vi "Flowmeter Final.vi"() -> ()   [LabVIEW 2018]
panel:
  in  "Induced EMF 5 (mV)":dbl(knob) scale=0.0..10.0
  in  "Induced EMF 4 (mV)":dbl(knob) scale=0.0..10.0
  in  "Induced EMF 3 (mV)":dbl(knob) scale=0.0..10.0
  in  "Induced EMF 2 (mV)":dbl(knob) scale=0.0..10.0
  in  "Electromagnetic Flow Meter Graphs":u16(ring) items=["EMF Induced", "Magnetic FIeld", "Diameter of Pipe"]
  in  "Doppler Flow Meter Graphs":u16(ring) items=["Ultrasound Speed", "Theta", "Frequency"]
  in  "Speed of Sound in Fluid (m/s)":dbl(knob) scale=0.0..1000.0
  out "XY Graph":cluster{"Y":dbl[], "Y":dbl[]}[](graph)
  in  "Switch 2":bool
  out "?":bool
  out "Velocity":dbl(knob) scale=0.0..1000.0
  in  "Ultrasonic Mode Switch":bool
  in  "?":bool
  in  "Thickness of pipe (mm)":dbl(slide) scale=0.0..1000.0
  in  "Magnetic Field (mT)":dbl(knob) scale=0.0..1000.0
  in  "Induced EMF 1 (mV)":dbl(knob) scale=0.0..10.0
  in  "Angle":dbl(knob) scale=90.0..30.0
  in  "Frequency 1 (KHz)":dbl(knob) scale=0.0..1000.0
  in  "Frequency 2 (KHz)":dbl(knob) scale=0.0..1000.0
  in  "milliseconds to wait":dbl
  in  "?":bool
  # "Variation wrt Difference\n      in Frequency"
  # "Variation wrt Angle"
  # "Electromagnetic"
  # "Ultrasonic"
  # "Doppler Flow Meter"
  # "Transit Time"
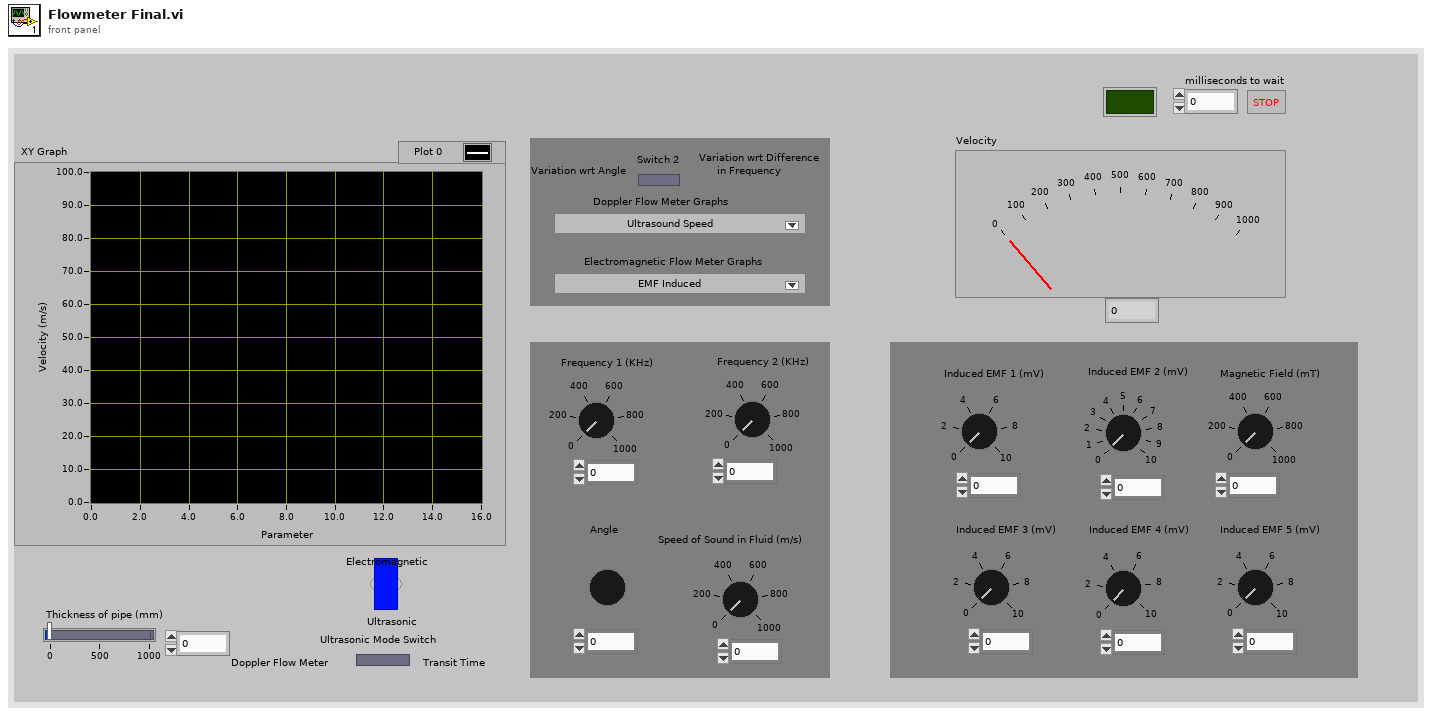
[diagram p1: front panel]
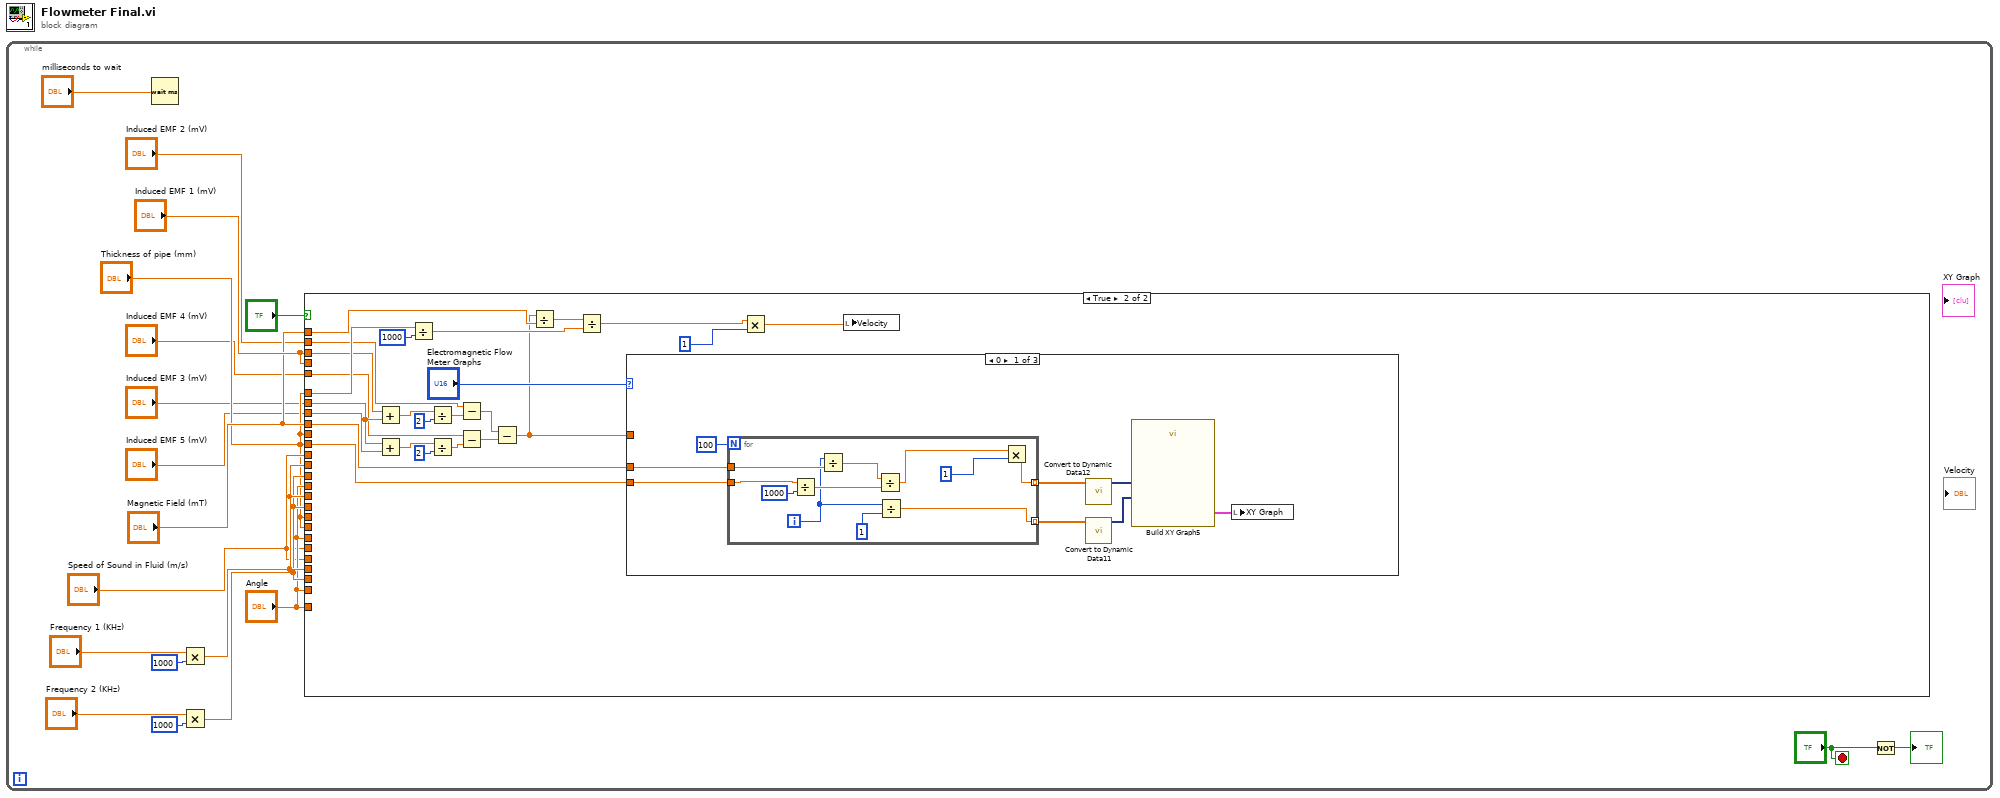
[diagram p0: block diagram]
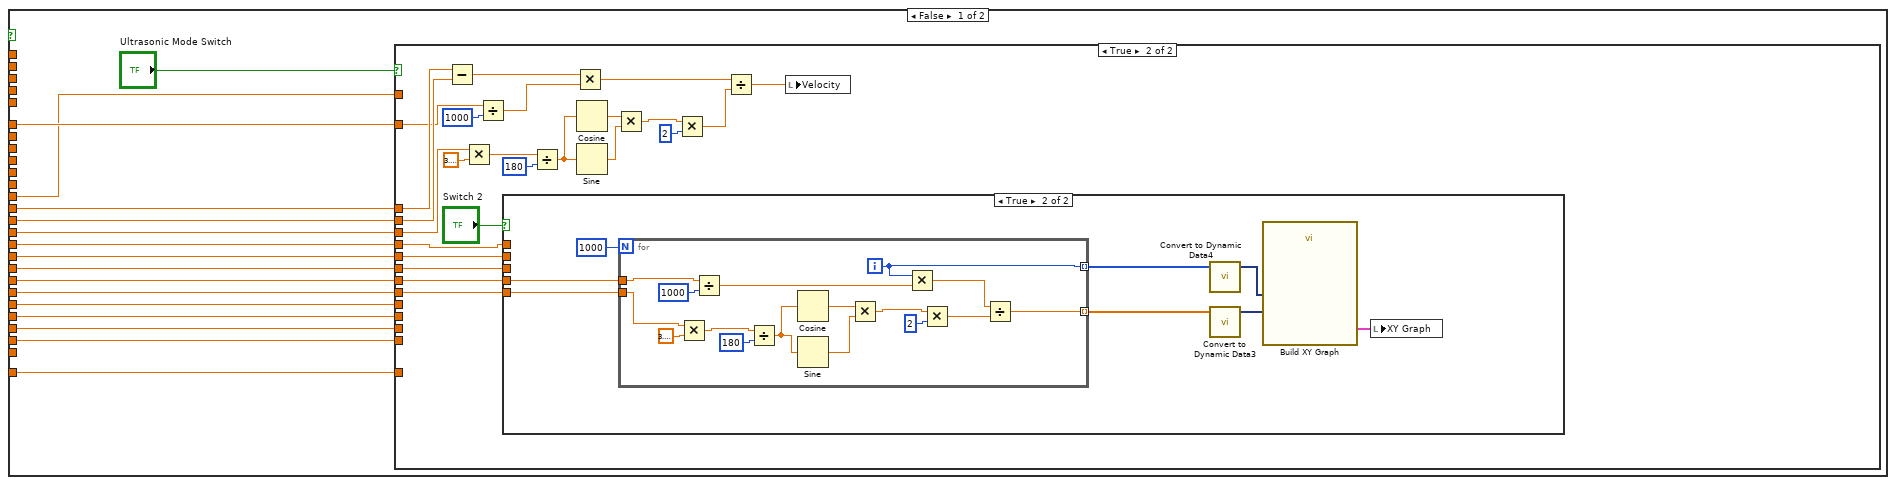
[diagram p2: hidden frame]
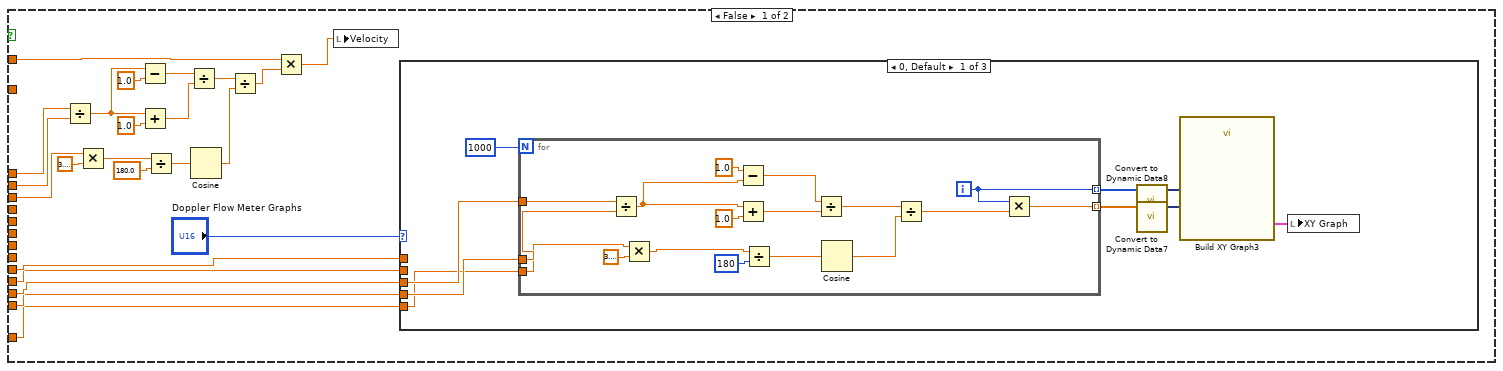
[diagram p3: hidden frame]
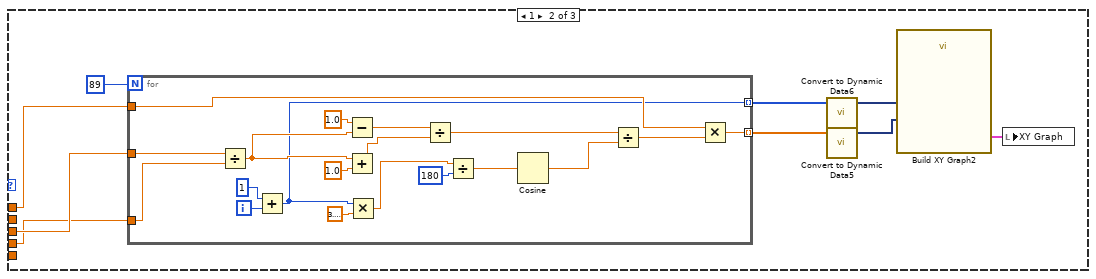
[diagram p4: hidden frame]
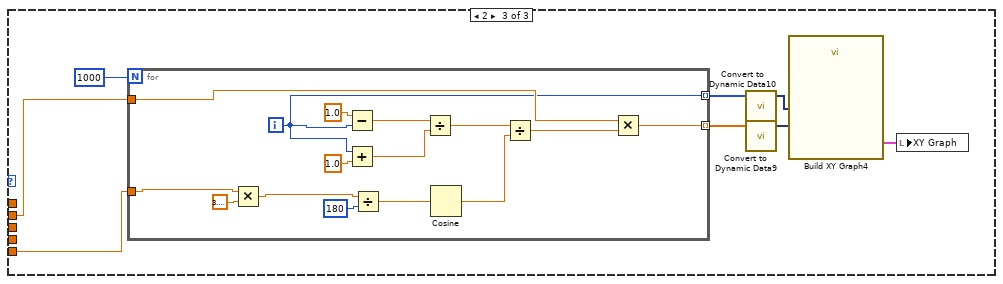
[diagram p5: hidden frame]
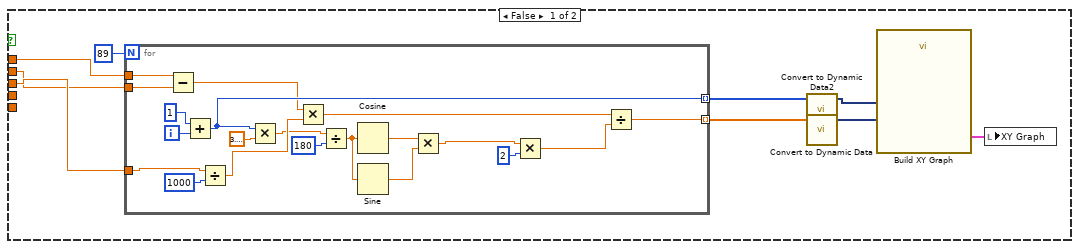
[diagram p6: hidden frame]
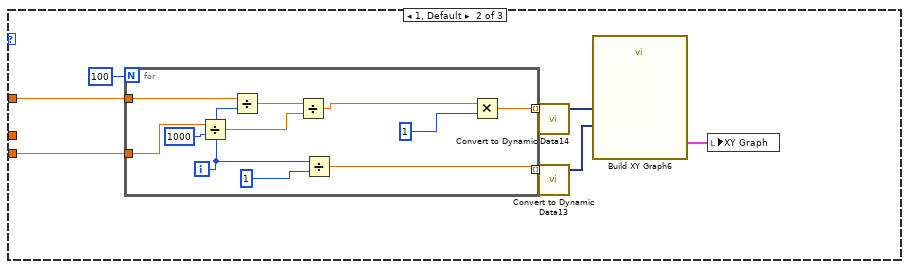
[diagram p7: hidden frame]
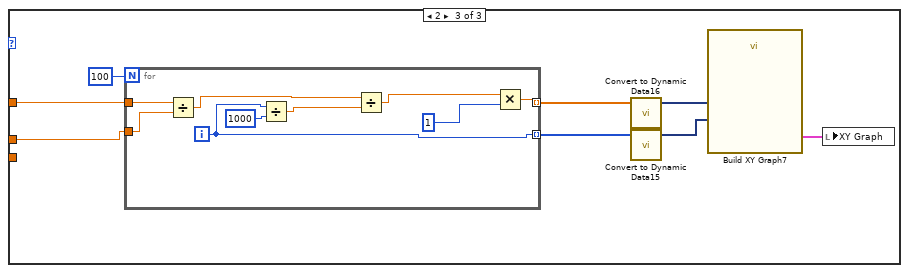
[diagram p8: hidden frame]
diagram:
  n1 = while {
    stop <- "?" stop-if-true
    n2 = Wait (ms)(milliseconds to wait="milliseconds to wait") -> ()  [unwired: 1 out]
    n3 = Multiply(x="Frequency 1 (KHz)", y=1000) -> (x*y=w11:dbl)
    n4 = Multiply(x="Frequency 2 (KHz)", y=1000) -> (x*y=w10:dbl)
    n5 = case shown="True" "?" {
      tunnel: "Angle" -> [w32 _]
      tunnel: "Thickness of pipe (mm)" -> [w33 w235]
      tunnel: w10 -> [w34 _]
      tunnel: w11 -> [w35 _]
      tunnel: "Angle" -> [_ _]
      tunnel: "Thickness of pipe (mm)" -> [_ _]
      tunnel: "Thickness of pipe (mm)" -> [w29 _]
      tunnel: w11 -> [w31 _]
      tunnel: w10 -> [w30 _]
      tunnel: "Induced EMF 1 (mV)" -> [_ w229]
      tunnel: "Magnetic Field (mT)" -> [_ w236]
      tunnel: "Thickness of pipe (mm)" -> [w27 _]
      tunnel: "Angle" -> [w26 _]
      tunnel: "Speed of Sound in Fluid (m/s)" -> [w25 _]
      tunnel: w11 -> [w24 _]
      tunnel: w10 -> [w23 _]
      tunnel: "Speed of Sound in Fluid (m/s)" -> [w22 _]
      tunnel: "Angle" -> [w21 _]
      tunnel: "Speed of Sound in Fluid (m/s)" -> [w20 _]
      tunnel: "Induced EMF 1 (mV)" -> [_ _]
      tunnel: "Magnetic Field (mT)" -> [_ w232]
      tunnel: "Thickness of pipe (mm)" -> [_ w231]
      tunnel: "Induced EMF 2 (mV)" -> [_ w220]
      tunnel: "Induced EMF 3 (mV)" -> [_ w228]
      tunnel: "Induced EMF 5 (mV)" -> [_ w227]
      tunnel: "Induced EMF 4 (mV)" -> [_ w219]
      frame False {
        n6 = case shown="True" "Ultrasonic Mode Switch" {
          tunnel: w35 -> [w46 w146]
          tunnel: w34 -> [w45 w145]
          tunnel: w33 -> [_ w144]
          tunnel: w32 -> [w44 w143]
          tunnel: w31 -> [_ w142]
          tunnel: w30 -> [_ w141]
          tunnel: w29 -> [_ w140]
          tunnel: w27 -> [_ w138]
          tunnel: w26 -> [_ w137]
          tunnel: w25 -> [w43 _]
          tunnel: w24 -> [w40 _]
          tunnel: w23 -> [w39 _]
          tunnel: w22 -> [w38 _]
          tunnel: w21 -> [w37 _]
          tunnel: w20 -> [w36 _]
          frame False {
            n7 = Divide(x=w46, y=w45) -> (x/y=w48:dbl)
            n8 = Multiply(x=w44, y=3.141592653589793) -> (x*y=w52:dbl)
            n9 = Subtract(x=w48, y=1.0 ("x")) -> (x-y=w57:dbl)
            n10 = Add(x=w48, y=1.0) -> (x+y=w56:dbl)
            n11 = Divide(x=w52, y=180.0) -> (x/y=w51:dbl)
            n12 = Divide(x=w57, y=w56) -> (x/y=w55:dbl)
            n13 = Cosine(x=w51) -> (cos(x)=w53:dbl)
            n14 = Divide(x=w55, y=w53) -> (x/y=w54:dbl)
            n15 = Multiply(x=w43, y=w54) -> (x*y=w42:dbl)
            n16 = local write "Velocity"(w42) -> ()
            n17 = case shown="0, Default" "Doppler Flow Meter Graphs" {
              tunnel: w40 -> [w62 w92 _]
              tunnel: w39 -> [w61 w91 _]
              tunnel: w38 -> [_ w90 _]
              tunnel: w37 -> [w60 _ w115]
              tunnel: w36 -> [_ _ w114]
              frame 0, Default {
                n18 = for {
                  N: 1000 -> [_]
                  tunnel: w62 -> [w77]
                  tunnel: w61 -> [w76]
                  tunnel: [w75] -> w63 mode=indexing
                  tunnel: [w68] -> w64 mode=indexing
                  tunnel: w60 -> [w69]
                  i -> [w68]
                  n19 = Divide(x=w77, y=w76) -> (x/y=w70:dbl)
                  n20 = Multiply(x=w69, y=3.141592653589793) -> (x*y=w74:dbl)
                  n21 = Subtract(x=1.0, y=w70) -> (x-y=w82:dbl)
                  n22 = Add(x=w70, y=1.0) -> (x+y=w81:dbl)
                  n23 = Divide(x=w74, y=180) -> (x/y=w71:dbl)
                  n24 = Divide(x=w82, y=w81) -> (x/y=w80:dbl)
                  n25 = Cosine(x=w71) -> (cos(x)=w78:dbl)
                  n26 = Divide(x=w80, y=w78) -> (x/y=w79:dbl)
                  n27 = Multiply(x=w68, y=w79) -> (x*y=w75:dbl)
                }
                n28 = call "Convert to Dynamic Data8"("Array"=w64) -> ("Dynamic Data Type"=w66:dynamicdata)  [unwired: 3 in]
                n29 = call "Convert to Dynamic Data7"("Array"=w63) -> ("Dynamic Data Type"=w65:dynamicdata)  [unwired: 3 in]
                n30 = call "Build XY Graph3"("Y Input"=w65, "X Input"=w66) -> ("XY Graph"=w59:cluster{"X":dbl[], "Y":dbl[]}[])  [unwired: 8 in, 1 out]
                n31 = local write "XY Graph"(w59) -> ()
              }
              frame 1 {
                n32 = for {
                  N: 89 -> [_]
                  tunnel: w92 -> [w105]
                  tunnel: w91 -> [w104]
                  tunnel: [w103] -> w86 mode=indexing
                  tunnel: [w94] -> w87 mode=indexing
                  tunnel: w90 -> [w95]
                  i -> [w102]
                  n33 = Divide(x=w105, y=w104) -> (x/y=w96:dbl)
                  n34 = Add(x=1, y=w102) -> (x+y=w94:i32)
                  n35 = Subtract(x=1.0, y=w96) -> (x-y=w110:dbl)
                  n36 = Add(x=w96, y=1.0) -> (x+y=w109:dbl)
                  n37 = Multiply(x=w94, y=3.141592653589793) -> (x*y=w100:dbl)
                  n38 = Divide(x=w110, y=w109) -> (x/y=w108:dbl)
                  n39 = Divide(x=w100, y=180) -> (x/y=w97:dbl)
                  n40 = Cosine(x=w97) -> (cos(x)=w106:dbl)
                  n41 = Divide(x=w108, y=w106) -> (x/y=w107:dbl)
                  n42 = Multiply(x=w95, y=w107) -> (x*y=w103:dbl)
                }
                n43 = call "Convert to Dynamic Data6"("Array"=w87) -> ("Dynamic Data Type"=w89:dynamicdata)  [unwired: 3 in]
                n44 = call "Convert to Dynamic Data5"("Array"=w86) -> ("Dynamic Data Type"=w88:dynamicdata)  [unwired: 3 in]
                n45 = call "Build XY Graph2"("Y Input"=w88, "X Input"=w89) -> ("XY Graph"=w85:cluster{"X":dbl[], "Y":dbl[]}[])  [unwired: 8 in, 1 out]
                n46 = local write "XY Graph"(w85) -> ()
              }
              frame 2 {
                n47 = for {
                  N: 1000 -> [_]
                  tunnel: [w128] -> w116 mode=indexing
                  tunnel: [w121] -> w117 mode=indexing
                  tunnel: w115 -> [w123]
                  tunnel: w114 -> [w122]
                  i -> [w121]
                  n48 = Multiply(x=w123, y=3.141592653589793) -> (x*y=w127:dbl)
                  n49 = Subtract(x=1.0, y=w121) -> (x-y=w133:dbl)
                  n50 = Add(x=w121, y=1.0) -> (x+y=w132:dbl)
                  n51 = Divide(x=w127, y=180) -> (x/y=w124:dbl)
                  n52 = Divide(x=w133, y=w132) -> (x/y=w131:dbl)
                  n53 = Cosine(x=w124) -> (cos(x)=w129:dbl)
                  n54 = Divide(x=w131, y=w129) -> (x/y=w130:dbl)
                  n55 = Multiply(x=w122, y=w130) -> (x*y=w128:dbl)
                }
                n56 = call "Convert to Dynamic Data10"("Array"=w117) -> ("Dynamic Data Type"=w119:dynamicdata)  [unwired: 3 in]
                n57 = call "Convert to Dynamic Data9"("Array"=w116) -> ("Dynamic Data Type"=w118:dynamicdata)  [unwired: 3 in]
                n58 = call "Build XY Graph4"("Y Input"=w118, "X Input"=w119) -> ("XY Graph"=w113:cluster{"X":dbl[], "Y":dbl[]}[])  [unwired: 8 in, 1 out]
                n59 = local write "XY Graph"(w113) -> ()
              }
            }
          }
          frame True {
            n60 = Subtract(x=w146, y=w145) -> (x-y=w147:dbl)
            n61 = Multiply(x=w143, y=3.141592653589793) -> (x*y=w157:dbl)
            n62 = Divide(x=w144, y=1000) -> (x/y=w148:dbl)
            n63 = case shown="True" "Switch 2" {
              tunnel: w137 -> [_ w191]
              tunnel: w138 -> [_ w190]
              tunnel: w140 -> [w163 _]
              tunnel: w142 -> [w162 _]
              tunnel: w141 -> [w161 _]
              frame False {
                n64 = for {
                  N: 89 -> [_]
                  tunnel: w163 -> [w176]
                  tunnel: w162 -> [w174]
                  tunnel: [w170] -> w164 mode=indexing
                  tunnel: [w175] -> w165 mode=indexing
                  tunnel: w161 -> [w173]
                  i -> [w172]
                  n65 = Subtract(x=w174, y=w173) -> (x-y=w169:dbl)
                  n66 = Add(x=1, y=w172) -> (x+y=w170:i32)
                  n67 = Divide(x=w176, y=1000) -> (x/y=w188:dbl)
                  n68 = Multiply(x=w170, y=3.141592653589793) -> (x*y=w181:dbl)
                  n69 = Multiply(x=w169, y=w188) -> (x*y=w186:dbl)
                  n70 = Divide(x=w181, y=180) -> (x/y=w182:dbl)
                  n71 = Cosine(x=w182) -> (cos(x)=w183:dbl)
                  n72 = Sine(x=w182) -> (sin(x)=w184:dbl)
                  n73 = Multiply(x=w183, y=w184) -> (x*y=w185:dbl)
                  n74 = Multiply(x=w185, y=2) -> (x*y=w187:dbl)
                  n75 = Divide(x=w186, y=w187) -> (x/y=w175:dbl)
                }
                n76 = call "Convert to Dynamic Data2"("Array"=w164) -> ("Dynamic Data Type"=w166:dynamicdata)  [unwired: 3 in]
                n77 = call "Convert to Dynamic Data"("Array"=w165) -> ("Dynamic Data Type"=w167:dynamicdata)  [unwired: 3 in]
                n78 = call "Build XY Graph"("Y Input"=w167, "X Input"=w166) -> ("XY Graph"=w160:cluster{"X":dbl[], "Y":dbl[]}[])  [unwired: 8 in, 1 out]
                n79 = local write "XY Graph"(w160) -> ()
              }
              frame True {
                n80 = for {
                  N: 1000 -> [_]
                  tunnel: w190 -> [w200]
                  tunnel: w191 -> [w199]
                  tunnel: [w197] -> w192 mode=indexing
                  tunnel: [w198] -> w193 mode=indexing
                  i -> [w197]
                  n81 = Multiply(x=w199, y=3.141592653589793) -> (x*y=w205:dbl)
                  n82 = Divide(x=w200, y=1000) -> (x/y=w212:dbl)
                  n83 = Divide(x=w205, y=180) -> (x/y=w206:dbl)
                  n84 = Cosine(x=w206) -> (cos(x)=w207:dbl)
                  n85 = Sine(x=w206) -> (sin(x)=w208:dbl)
                  n86 = Multiply(x=w207, y=w208) -> (x*y=w209:dbl)
                  n87 = Multiply(x=w197, y=w212) -> (x*y=w210:dbl)
                  n88 = Multiply(x=w209, y=2) -> (x*y=w211:dbl)
                  n89 = Divide(x=w210, y=w211) -> (x/y=w198:dbl)
                }
                n90 = call "Convert to Dynamic Data4"("Array"=w192) -> ("Dynamic Data Type"=w194:dynamicdata)  [unwired: 3 in]
                n91 = call "Convert to Dynamic Data3"("Array"=w193) -> ("Dynamic Data Type"=w195:dynamicdata)  [unwired: 3 in]
                n92 = call "Build XY Graph"("Y Input"=w195, "X Input"=w194) -> ("XY Graph"=w189:cluster{"X":dbl[], "Y":dbl[]}[])  [unwired: 8 in, 1 out]
                n93 = local write "XY Graph"(w189) -> ()
              }
            }
            n94 = Divide(x=w157, y=180) -> (x/y=w155:dbl)
            n95 = Multiply(x=w147, y=w148) -> (x*y=w151:dbl)
            n96 = Cosine(x=w155) -> (cos(x)=w154:dbl)
            n97 = Sine(x=w155) -> (sin(x)=w153:dbl)
            n98 = Multiply(x=w154, y=w153) -> (x*y=w152:dbl)
            n99 = Multiply(x=w152, y=2) -> (x*y=w150:dbl)
            n100 = Divide(x=w151, y=w150) -> (x/y=w136:dbl)
            n101 = local write "Velocity"(w136) -> ()
          }
        }
      }
      frame True {
        n102 = Add(x=w229, y=w228) -> (x+y=w226:dbl)
        n103 = Add(x=w228, y=w227) -> (x+y=w225:dbl)
        n104 = Divide(x=w235, y=1000) -> (x/y=w233:dbl)
        n105 = Divide(x=w226, y=2) -> (x/y=w224:dbl)
        n106 = Divide(x=w225, y=2) -> (x/y=w223:dbl)
        n107 = Subtract(x=w220, y=w224) -> (x-y=w217:dbl)
        n108 = Subtract(x=w219, y=w223) -> (x-y=w216:dbl)
        n109 = Subtract(x=w217, y=w216) -> (x-y=w218:dbl)
        n110 = Divide(x=w218, y=w236) -> (x/y=w234:dbl)
        n111 = Divide(x=w234, y=w233) -> (x/y=w215:dbl)
        n112 = case shown="0" "Electromagnetic Flow Meter Graphs" {
          tunnel: w218 -> [_ w260 w279]
          tunnel: w232 -> [w245 _ w278]
          tunnel: w231 -> [w240 w259 _]
          frame 0 {
            n113 = for {
              N: 100 -> [_]
              tunnel: [w250] -> w242 mode=indexing
              tunnel: w245 -> [w253]
              tunnel: [w246] -> w241 mode=indexing
              tunnel: w240 -> [w252]
              i -> [w247]
              n114 = Divide(x=w252, y=1000) -> (x/y=w254:dbl)
              n115 = Divide(x=w247, y=w253) -> (x/y=w255:dbl)
              n116 = Divide(x=w255, y=w254) -> (x/y=w249:dbl)
              n117 = Divide(x=w247, y=1) -> (x/y=w246:dbl)
              n118 = Multiply(x=w249, y=1) -> (x*y=w250:dbl)
            }
            n119 = call "Convert to Dynamic Data12"("Array"=w242) -> ("Dynamic Data Type"=w244:dynamicdata)  [unwired: 3 in]
            n120 = call "Convert to Dynamic Data11"("Array"=w241) -> ("Dynamic Data Type"=w243:dynamicdata)  [unwired: 3 in]
            n121 = call "Build XY Graph5"("Y Input"=w243, "X Input"=w244) -> ("XY Graph"=w238:cluster{"X":dbl[], "Y":dbl[]}[])  [unwired: 8 in, 1 out]
            n122 = local write "XY Graph"(w238) -> ()
          }
          frame 1, Default {
            n123 = for {
              N: 100 -> [_]
              tunnel: [w268] -> w261 mode=indexing
              tunnel: w260 -> [w272]
              tunnel: w259 -> [w271]
              tunnel: [w265] -> w258 mode=indexing
              i -> [w267]
              n124 = Divide(x=w271, y=1000) -> (x/y=w273:dbl)
              n125 = Divide(x=w272, y=w267) -> (x/y=w274:dbl)
              n126 = Divide(x=w274, y=w273) -> (x/y=w269:dbl)
              n127 = Divide(x=w267, y=1) -> (x/y=w265:dbl)
              n128 = Multiply(x=w269, y=1) -> (x*y=w268:dbl)
            }
            n129 = call "Convert to Dynamic Data14"("Array"=w261) -> ("Dynamic Data Type"=w263:dynamicdata)  [unwired: 3 in]
            n130 = call "Convert to Dynamic Data13"("Array"=w258) -> ("Dynamic Data Type"=w262:dynamicdata)  [unwired: 3 in]
            n131 = call "Build XY Graph6"("Y Input"=w262, "X Input"=w263) -> ("XY Graph"=w257:cluster{"X":dbl[], "Y":dbl[]}[])  [unwired: 8 in, 1 out]
            n132 = local write "XY Graph"(w257) -> ()
          }
          frame 2 {
            n133 = for {
              N: 100 -> [_]
              tunnel: [w285] -> w280 mode=indexing
              tunnel: w279 -> [w290]
              tunnel: w278 -> [w289]
              tunnel: [w284] -> w277 mode=indexing
              i -> [w284]
              n134 = Divide(x=w290, y=w289) -> (x/y=w291:dbl)
              n135 = Divide(x=w284, y=1000) -> (x/y=w288:dbl)
              n136 = Divide(x=w291, y=w288) -> (x/y=w286:dbl)
              n137 = Multiply(x=w286, y=1) -> (x*y=w285:dbl)
            }
            n138 = call "Convert to Dynamic Data16"("Array"=w280) -> ("Dynamic Data Type"=w281:dynamicdata)  [unwired: 3 in]
            n139 = call "Convert to Dynamic Data15"("Array"=w277) -> ("Dynamic Data Type"=w282:dynamicdata)  [unwired: 3 in]
            n140 = call "Build XY Graph7"("Y Input"=w282, "X Input"=w281) -> ("XY Graph"=w276:cluster{"X":dbl[], "Y":dbl[]}[])  [unwired: 8 in, 1 out]
            n141 = local write "XY Graph"(w276) -> ()
          }
        }
        n142 = Multiply(x=w215, y=1) -> (x*y=w213:dbl)
        n143 = local write "Velocity"(w213) -> ()
      }
    }
    n144 = Not(x="?") -> (.not. x?=→"?":bool)
  }
